vi "Exp_SetTemplate.vi"(8 "error in (no error)":errorcluster, 10 "Setting":i32, 11 "LightField Automation in":refnum<class "LightField Automation.lvclass">) -> (0 "error out":errorcluster, 3 "LightField Automation out":refnum<class "LightField Automation.lvclass">)   [LabVIEW 2019, in "LightField Automation.lvclass"]
uses:
  LightField Automation.lvclass
  C:/Program Files/Princeton Instruments/LightField/PrincetonInstruments.LightFieldAddInSupportServices.dll
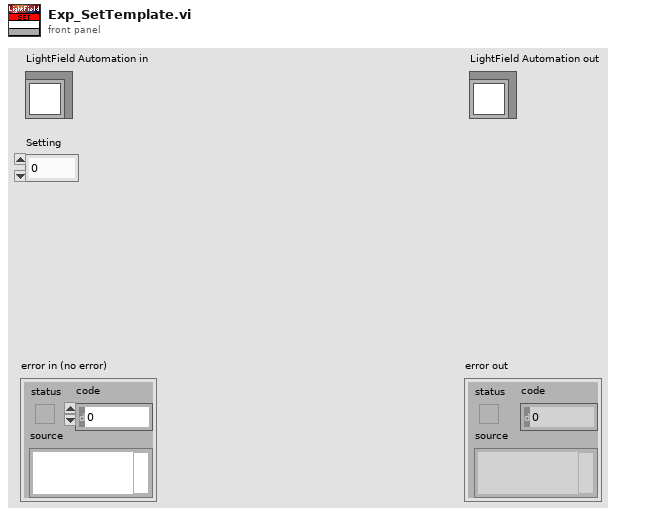
[diagram p1: front panel]
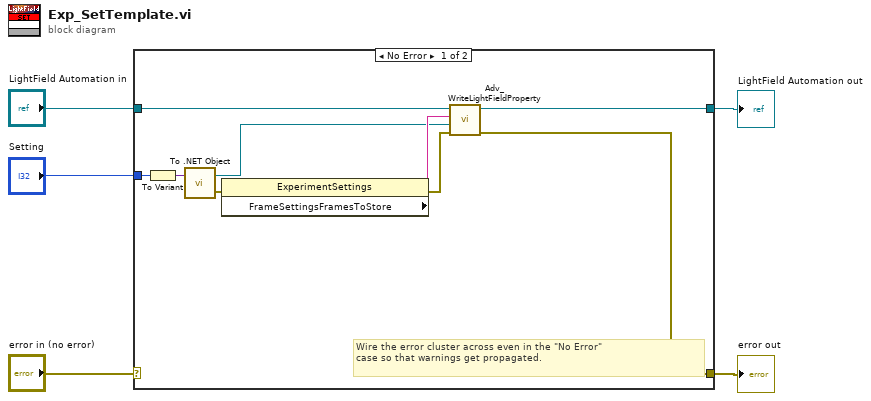
[diagram p0: block diagram]
diagram:
  n1 = case shown="No Error" "error in (no error)" {
    selector: "error in (no error)" -> [_ w16]
    tunnel: [w6 w16] -> w4
    tunnel: [w10 w15] -> w2
    tunnel: "LightField Automation in" -> [w11 w15]
    tunnel: "Setting" -> [w14 _]
    frame No Error {
      # "Wire the error cluster across even in the \"No Error\"\ncase so that warnings get propagated."
      n2 = To Variant(anything=w14) -> (Variant=w13:variant)
      n3 = call <vilib>:"To .NET Object.vi"("anything"=w13) -> ("error out"=w12:errorcluster, ".NET object"=w8:refnum<k24>)  [unwired: 1 in]
      n4 = property class="ExperimentSettings"(error in=w12) -> (error out=w7:errorcluster, "FrameSettingsFramesToStore"=w9:string)  [unwired: 1 in, 1 out]
      n5 = call "Adv_WriteLightFieldProperty.vi"("error in (no error)"=w7, "value"=w8, "setting"=w9, "LightField Automation in"=w11) -> ("error out"=w6:errorcluster, "LightField Automation out"=w10:refnum<class "LightField Automation.lvclass">)  [unwired: 6 in]
    }
    frame Error {
    }
  }
  "error out" <- w4
  "LightField Automation out" <- w2
